vi "PCO_GetFirmwareInfo.vi"(8 "error in (no error)":errorcluster {"code" format="%x"}, 10 "wDeviceBlock":u16, 11 "ph":u64) -> (0 "error out":errorcluster {"code" format="%x"}, 1 "strFirmwareVersion":T1, 2 "ErrorMessage":i32 format="%x", 3 "ph out":u64)   [LabVIEW 2019, in "SDK.lvlib" / "GeneralCameraStatus.lvlib"]
doc: "<b>Description:</b>\nQuery firmware versions of all devices in the camera such as main microprocessor, main FPGA and coprocessors of the interface boards. Because the number of devices can exceed the number of information fields of the PCO_FW_Vers structure additional blocks of information can be requested using the wDeviceBlock parameter. The first call should be made with wDeviceBlock parameter set to 0. On return the wDeviceNum parameter of the PCO_FW_Vers will be filled with the number of all installed devices in the camera. Up to this number, each Device structure will contain the firmware information for a particular device. Further calls with increasing wDeviceBlock parameter might be necessary to get all available firmware versions.\n\n<b>Supported camera type:</b>\nAll cameras\n\n<b>Descriptor dependency:</b>\nNone"
uses:
  GeneralCameraStatus.lvlib
  Structures/Structures.lvlib
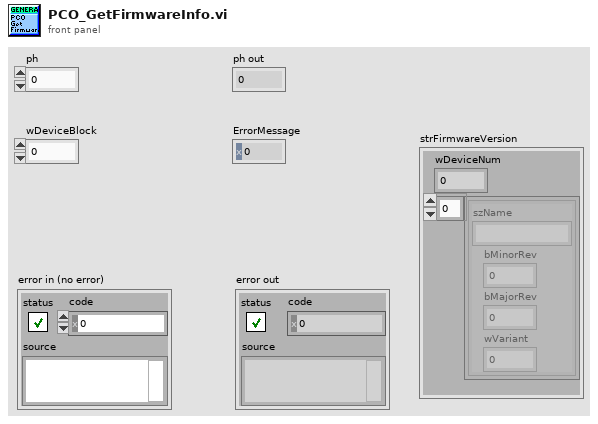
[diagram p1: front panel]
types:
  T1 = cluster{"wDeviceNum":u16, cluster{"szName":string, "bMinorRev":u8, "bMajorRev":u8, "wVariant":u16}[]}
  T2 = cluster{"wDeviceNum":u16, "PCO_SC2_Firmware_DESC":cluster{"szName":string, "bMinorRev":u8, "bMajorRev":u8, "wVariant":u16}[]}
  T3 = cluster{"wDeviceNum":u16, "PCO_SC2_Firmware_DESC":cluster{"PCO_SC2_FW_Desc_Raw":cluster{"szName":cluster{u8, u8, u8, u8, u8, u8, u8, u8, u8, u8, u8, u8, u8, u8, u8, u8}, "bMinorRev":u8, "bMajorRev":u8, "wVariant":u16, "zzwDummy":cluster{u16, u16, u16, u16, u16, u16, u16, u16, u16, u16, u16, u16, u16, u16, u16, u16, u16, u16, u16, u16, u16, u16}}, "PCO_SC2_FW_Desc_Raw":cluster{"szName":cluster{u8, u8, u8, u8, u8, u8, u8, u8, u8, u8, u8, u8, u8, u8, u8, u8}, "bMinorRev":u8, "bMajorRev":u8, "wVariant":u16, "zzwDummy":cluster{u16, u16, u16, u16, u16, u16, u16, u16, u16, u16, u16, u16, u16, u16, u16, u16, u16, u16, u16, u16, u16, u16}}, "PCO_SC2_FW_Desc_Raw":cluster{"szName":cluster{u8, u8, u8, u8, u8, u8, u8, u8, u8, u8, u8, u8, u8, u8, u8, u8}, "bMinorRev":u8, "bMajorRev":u8, "wVariant":u16, "zzwDummy":cluster{u16, u16, u16, u16, u16, u16, u16, u16, u16, u16, u16, u16, u16, u16, u16, u16, u16, u16, u16, u16, u16, u16}}, "PCO_SC2_FW_Desc_Raw":cluster{"szName":cluster{u8, u8, u8, u8, u8, u8, u8, u8, u8, u8, u8, u8, u8, u8, u8, u8}, "bMinorRev":u8, "bMajorRev":u8, "wVariant":u16, "zzwDummy":cluster{u16, u16, u16, u16, u16, u16, u16, u16, u16, u16, u16, u16, u16, u16, u16, u16, u16, u16, u16, u16, u16, u16}}, "PCO_SC2_FW_Desc_Raw":cluster{"szName":cluster{u8, u8, u8, u8, u8, u8, u8, u8, u8, u8, u8, u8, u8, u8, u8, u8}, "bMinorRev":u8, "bMajorRev":u8, "wVariant":u16, "zzwDummy":cluster{u16, u16, u16, u16, u16, u16, u16, u16, u16, u16, u16, u16, u16, u16, u16, u16, u16, u16, u16, u16, u16, u16}}, "PCO_SC2_FW_Desc_Raw":cluster{"szName":cluster{u8, u8, u8, u8, u8, u8, u8, u8, u8, u8, u8, u8, u8, u8, u8, u8}, "bMinorRev":u8, "bMajorRev":u8, "wVariant":u16, "zzwDummy":cluster{u16, u16, u16, u16, u16, u16, u16, u16, u16, u16, u16, u16, u16, u16, u16, u16, u16, u16, u16, u16, u16, u16}}, "PCO_SC2_FW_Desc_Raw":cluster{"szName":cluster{u8, u8, u8, u8, u8, u8, u8, u8, u8, u8, u8, u8, u8, u8, u8, u8}, "bMinorRev":u8, "bMajorRev":u8, "wVariant":u16, "zzwDummy":cluster{u16, u16, u16, u16, u16, u16, u16, u16, u16, u16, u16, u16, u16, u16, u16, u16, u16, u16, u16, u16, u16, u16}}, "PCO_SC2_FW_Desc_Raw":cluster{"szName":cluster{u8, u8, u8, u8, u8, u8, u8, u8, u8, u8, u8, u8, u8, u8, u8, u8}, "bMinorRev":u8, "bMajorRev":u8, "wVariant":u16, "zzwDummy":cluster{u16, u16, u16, u16, u16, u16, u16, u16, u16, u16, u16, u16, u16, u16, u16, u16, u16, u16, u16, u16, u16, u16}}, "PCO_SC2_FW_Desc_Raw":cluster{"szName":cluster{u8, u8, u8, u8, u8, u8, u8, u8, u8, u8, u8, u8, u8, u8, u8, u8}, "bMinorRev":u8, "bMajorRev":u8, "wVariant":u16, "zzwDummy":cluster{u16, u16, u16, u16, u16, u16, u16, u16, u16, u16, u16, u16, u16, u16, u16, u16, u16, u16, u16, u16, u16, u16}}, "PCO_SC2_FW_Desc_Raw":cluster{"szName":cluster{u8, u8, u8, u8, u8, u8, u8, u8, u8, u8, u8, u8, u8, u8, u8, u8}, "bMinorRev":u8, "bMajorRev":u8, "wVariant":u16, "zzwDummy":cluster{u16, u16, u16, u16, u16, u16, u16, u16, u16, u16, u16, u16, u16, u16, u16, u16, u16, u16, u16, u16, u16, u16}}}}
  T4 = cluster{"PCO_SC2_FW_Desc_Raw":cluster{"szName":cluster{u8, u8, u8, u8, u8, u8, u8, u8, u8, u8, u8, u8, u8, u8, u8, u8}, "bMinorRev":u8, "bMajorRev":u8, "wVariant":u16, "zzwDummy":cluster{u16, u16, u16, u16, u16, u16, u16, u16, u16, u16, u16, u16, u16, u16, u16, u16, u16, u16, u16, u16, u16, u16}}, "PCO_SC2_FW_Desc_Raw":cluster{"szName":cluster{u8, u8, u8, u8, u8, u8, u8, u8, u8, u8, u8, u8, u8, u8, u8, u8}, "bMinorRev":u8, "bMajorRev":u8, "wVariant":u16, "zzwDummy":cluster{u16, u16, u16, u16, u16, u16, u16, u16, u16, u16, u16, u16, u16, u16, u16, u16, u16, u16, u16, u16, u16, u16}}, "PCO_SC2_FW_Desc_Raw":cluster{"szName":cluster{u8, u8, u8, u8, u8, u8, u8, u8, u8, u8, u8, u8, u8, u8, u8, u8}, "bMinorRev":u8, "bMajorRev":u8, "wVariant":u16, "zzwDummy":cluster{u16, u16, u16, u16, u16, u16, u16, u16, u16, u16, u16, u16, u16, u16, u16, u16, u16, u16, u16, u16, u16, u16}}, "PCO_SC2_FW_Desc_Raw":cluster{"szName":cluster{u8, u8, u8, u8, u8, u8, u8, u8, u8, u8, u8, u8, u8, u8, u8, u8}, "bMinorRev":u8, "bMajorRev":u8, "wVariant":u16, "zzwDummy":cluster{u16, u16, u16, u16, u16, u16, u16, u16, u16, u16, u16, u16, u16, u16, u16, u16, u16, u16, u16, u16, u16, u16}}, "PCO_SC2_FW_Desc_Raw":cluster{"szName":cluster{u8, u8, u8, u8, u8, u8, u8, u8, u8, u8, u8, u8, u8, u8, u8, u8}, "bMinorRev":u8, "bMajorRev":u8, "wVariant":u16, "zzwDummy":cluster{u16, u16, u16, u16, u16, u16, u16, u16, u16, u16, u16, u16, u16, u16, u16, u16, u16, u16, u16, u16, u16, u16}}, "PCO_SC2_FW_Desc_Raw":cluster{"szName":cluster{u8, u8, u8, u8, u8, u8, u8, u8, u8, u8, u8, u8, u8, u8, u8, u8}, "bMinorRev":u8, "bMajorRev":u8, "wVariant":u16, "zzwDummy":cluster{u16, u16, u16, u16, u16, u16, u16, u16, u16, u16, u16, u16, u16, u16, u16, u16, u16, u16, u16, u16, u16, u16}}, "PCO_SC2_FW_Desc_Raw":cluster{"szName":cluster{u8, u8, u8, u8, u8, u8, u8, u8, u8, u8, u8, u8, u8, u8, u8, u8}, "bMinorRev":u8, "bMajorRev":u8, "wVariant":u16, "zzwDummy":cluster{u16, u16, u16, u16, u16, u16, u16, u16, u16, u16, u16, u16, u16, u16, u16, u16, u16, u16, u16, u16, u16, u16}}, "PCO_SC2_FW_Desc_Raw":cluster{"szName":cluster{u8, u8, u8, u8, u8, u8, u8, u8, u8, u8, u8, u8, u8, u8, u8, u8}, "bMinorRev":u8, "bMajorRev":u8, "wVariant":u16, "zzwDummy":cluster{u16, u16, u16, u16, u16, u16, u16, u16, u16, u16, u16, u16, u16, u16, u16, u16, u16, u16, u16, u16, u16, u16}}, "PCO_SC2_FW_Desc_Raw":cluster{"szName":cluster{u8, u8, u8, u8, u8, u8, u8, u8, u8, u8, u8, u8, u8, u8, u8, u8}, "bMinorRev":u8, "bMajorRev":u8, "wVariant":u16, "zzwDummy":cluster{u16, u16, u16, u16, u16, u16, u16, u16, u16, u16, u16, u16, u16, u16, u16, u16, u16, u16, u16, u16, u16, u16}}, "PCO_SC2_FW_Desc_Raw":cluster{"szName":cluster{u8, u8, u8, u8, u8, u8, u8, u8, u8, u8, u8, u8, u8, u8, u8, u8}, "bMinorRev":u8, "bMajorRev":u8, "wVariant":u16, "zzwDummy":cluster{u16, u16, u16, u16, u16, u16, u16, u16, u16, u16, u16, u16, u16, u16, u16, u16, u16, u16, u16, u16, u16, u16}}}
  T5 = cluster{"szName":string, "bMinorRev":u8, "bMajorRev":u8, "wVariant":u16}
  T6 = cluster{"szName":cluster{u8, u8, u8, u8, u8, u8, u8, u8, u8, u8, u8, u8, u8, u8, u8, u8}, "bMinorRev":u8, "bMajorRev":u8, "wVariant":u16, "zzwDummy":cluster{u16, u16, u16, u16, u16, u16, u16, u16, u16, u16, u16, u16, u16, u16, u16, u16, u16, u16, u16, u16, u16, u16}}[]
  T7 = cluster{"szName":string, "bMinorRev":u8, "bMajorRev":u8, "wVariant":u16}[]
  T8 = cluster{u8, u8, u8, u8, u8, u8, u8, u8, u8, u8, u8, u8, u8, u8, u8, u8}
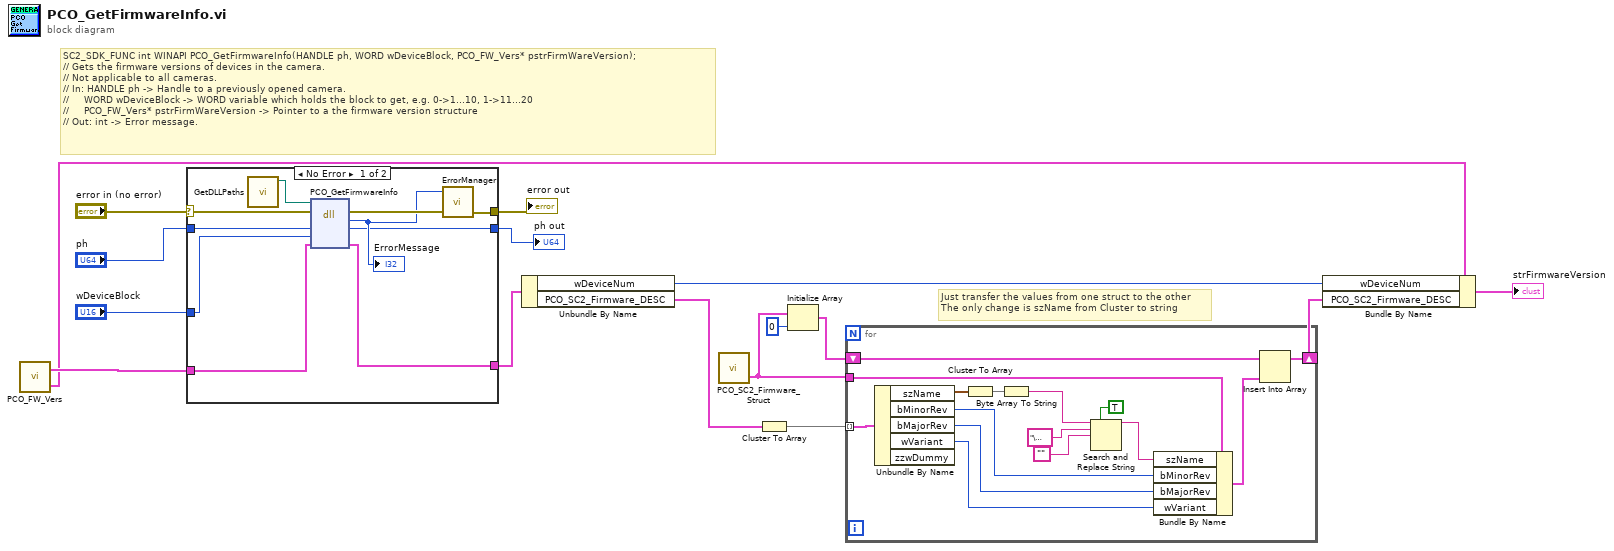
[diagram p0: block diagram]
diagram:
  # "Just transfer the values from one struct to the other\nThe only change is szName from Cluster to string"
  # "SC2_SDK_FUNC int WINAPI PCO_GetFirmwareInfo(HANDLE ph, WORD wDeviceBlock, PCO_FW_Vers* pstrFirmWareVersion);\n// Gets the firmware versions of devices in the camera.\n// Not applicable to all cameras.\n// In: HANDLE ph -> Handle to a previously opened camera.\n//     WORD wDeviceBlock -> WORD variable which holds the block to get, e.g. 0->1...10, 1->11...20\n//     PCO_FW_Vers* pstrFirmWareVersion -> Pointer to a the firmware version structure\n// Out: int -> Error message."
  n1 = call "PCO_FW_Vers.vi"() -> ("PCO_FW_Vers"=w2:T2, "PCO_FW_Vers_Raw"=w3:T3)  [unwired: 4 in, 2 out]
  n2 = case shown="No Error" "error in (no error)" {
    selector: "error in (no error)" -> [w26 w29]
    tunnel: [w23 w29] -> w16
    tunnel: "ph" -> [w25 w28]
    tunnel: [w21 w28] -> w13
    tunnel: w3 -> [w20 w27]
    tunnel: [w19 w27] -> w5
    tunnel: "wDeviceBlock" -> [w18 _]
    frame No Error {
      n3 = call "GetDLLPaths.vi"() -> ("SC2_Cam_Path"=w17:path)  [unwired: 8 in, 3 out]
      n4 = dll-call lib="?" fn="PCO_GetFirmwareInfo"(path in=w17, error in=w26, "ph"=w25, "wDeviceBlock"=w18, "pstrFirmWareVersion"=w20) -> (error out=w24:errorcluster, "return type"=w22:i32, "ph"=w21:u64, "pstrFirmWareVersion"=w19:T3)  [unwired: 2 in, 1 out]
      "ErrorMessage" <- w22
      n5 = call "ErrorManager.vi"("error in (no error)"=w24, "error code"=w22) -> ("error out"=w23:errorcluster)  [unwired: 2 in, 1 out]
    }
    frame Error {
    }
  }
  "error out" <- w16
  "ph out" <- w13
  n6 = Unbundle By Name(w5) -> ("wDeviceNum"=w7:u16, "PCO_SC2_Firmware_DESC"=w12:T4)
  n7 = call "PCO_SC2_Firmware_Struct.vi"() -> ("PCO_SC2_FW_Desc"=w9:T5)  [unwired: 4 in, 3 out]
  n8 = Cluster To Array(cluster=w12) -> (array=w11:T6)
  n9 = Initialize Array(w9, 0 ("dimension size")) -> (w8:T7)
  n10 = for {
    tunnel: w11 -> [w39] mode=indexing
    shift-right: [w38] -> w6
    shift-left: w8 -> [w36]
    tunnel: w9 -> [w35]
    n11 = Unbundle By Name(w39) -> ("szName"=w44:T8, "bMinorRev"=w42:u8, "bMajorRev"=w41:u8, "wVariant"=w40:u16)  [unwired: 1 out]
    n12 = Cluster To Array(cluster=w44) -> (array=w43:u8[])
    n13 = Byte Array To String(unsigned byte array=w43) -> (string=w31:string)
    n14 = Search and Replace String(replace all?=TRUE ("replace all? (F)"), input string=w31, search string="\u0000", replace string="" ("replace string (\"\")")) -> (result string=w30:string)  [unwired: 4 in, 3 out]
    n15 = Bundle By Name(cluster=w35, "szName"=w30, "bMinorRev"=w42, "bMajorRev"=w41, "wVariant"=w40) -> (w37:T5)
    n16 = Insert Into Array(array=w36, new element=w37) -> (w38:T7)  [unwired: 1 in]
  }
  n17 = Bundle By Name(cluster=w2, "wDeviceNum"=w7, "PCO_SC2_Firmware_DESC"=w6) -> (→"strFirmwareVersion":T2)
